vi "Construct Server Controller.vi"(8 "error in (no error)":errorcluster, 10 "Root Path":path) -> (0 "error out":errorcluster, 3 "Test Step Controller out":refnum<class "Server Controller.lvclass">)   [LabVIEW 2016, in "Server Controller.lvlib" / "Server Controller.lvclass"]
uses:
  Controller/Server Controller.lvclass
  \\Mac\Home/Documents/MAL-Framework/user.lib/Common Components/Controller/Controller.lvclass
  UI/Server UI.lvclass
  \\Mac\Home/Documents/MAL-Framework/user.lib/Common Components/User Interface/UI.lvclass
  Controller/Server Config.lvclass
  C:/Program Files (x86)/National Instruments/LabVIEW 2016/user.lib/Configuration Dialog Actor/Configuration.lvclass
  MAL-Framework/user.lib/Common Components/Controller/Controller.lvclass/Controller.ctl
  MAL-Framework/user.lib/Common Components/Controller/Accessors/Write Root Path.vi
  MAL-Framework/user.lib/Common Components/Controller/Controller.lvclass
  <userlib>/Configuration Dialog Actor/Configuration.lvclass
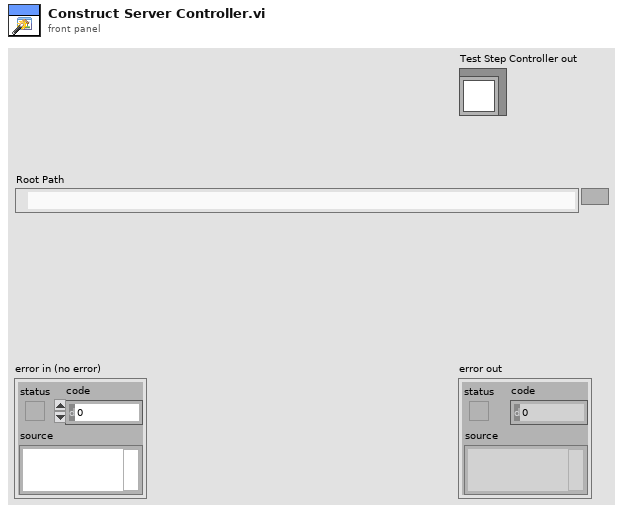
[diagram p1: front panel]
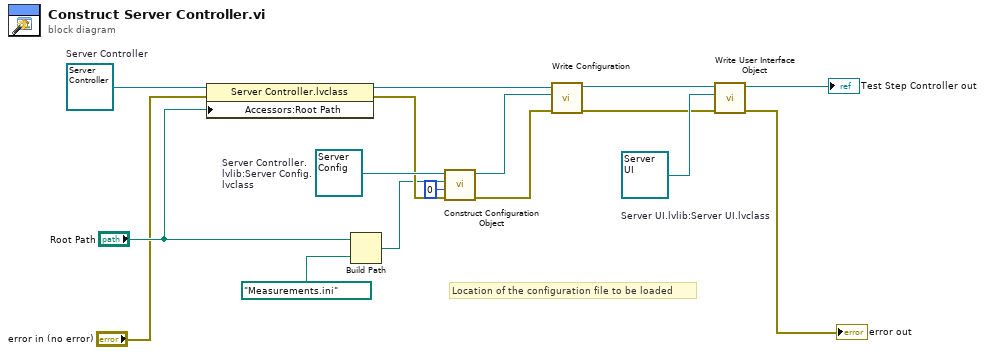
[diagram p0: block diagram]
diagram:
  w11 = refnum<class "Server Config.lvclass"> refnum  # Server Controller.lvlib:Server Config.lvclass
  w14 = refnum<class "Server UI.lvclass"> refnum  # Server UI.lvlib:Server UI.lvclass
  w7 = refnum<class "Server Controller.lvclass"> refnum  # Server Controller
  # "Location of the configuration file to be loaded"
  n1 = property class="Server Controller.lvclass"(reference=w7, error in="error in (no error)", "Accessors:Root Path"="Root Path") -> (reference out=w6:refnum<class "Server Controller.lvclass">, error out=w4:errorcluster)
  n2 = Build Path(base path="Root Path", name or relative path=path "Measurements.ini" ("VI Path")) -> (appended path=w1:path)
  n3 = call <userlib>:"Construct Configuration Object.vi"("error in (no error)"=w4, "Initial Category Selection"=0, "Configuration File Path"=w1, "Configuration in"=w11) -> ("error out"=w9:errorcluster, "Configuration out"=w10:refnum<class "Server Config.lvclass">)  [unwired: 4 in, 2 out]
  n4 = call "Write Configuration.vi"("error in (no error)"=w9, "Configuration.lvlib:Configuration.lvclass"=w10, "Controller in"=w6) -> ("error out"=w12:errorcluster, "Controller in"=w13:refnum<class "Server Controller.lvclass">)  [unwired: 7 in]
  n5 = call "Write User Interface Object.vi"("error in (no error)"=w12, "UI.lvclass"=w14, "UI Controller in"=w13) -> ("error out"=→"error out":errorcluster, "UI Controller out"=→"Test Step Controller out":refnum<class "Server Controller.lvclass">)  [unwired: 7 in]
